vi "Global Conveyor.vi"() -> ()   [LabVIEW 2019]
panel:
  in  "MoveIntake":bool
  in  "Intake":bool
  in  "Shoot":bool
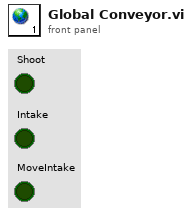
[diagram p1: front panel]
diagram:
